vi "Test Multiple Doors API.vi"() -> ()   [LabVIEW 2018]
uses:
  DoorInterface_interface/DoorInterface.lvclass
  Door/Door.lvclass
  Timed Door.lvclass
  Set Target Time (seconds).vi
panel:
  out "error out":errorcluster
  in  "Create New Door":bool
  in  "Door Type":enum32{"Door", "Timed Door"}(radio)
  in  "Timed Door Target Time (seconds)":dbl=5.0
  in  "Door Switches":enum32{"Open Door", "Close Door"}[](array[radio])
  out "Doors":u16[](array[ring])
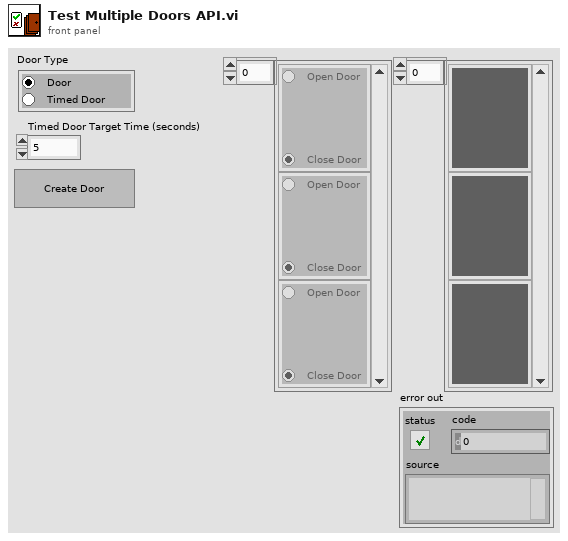
[diagram p1: front panel]
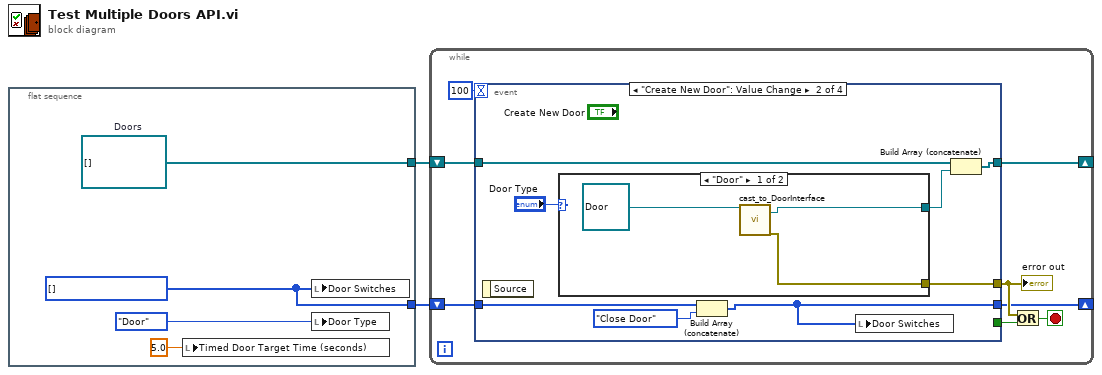
[diagram p0: block diagram]
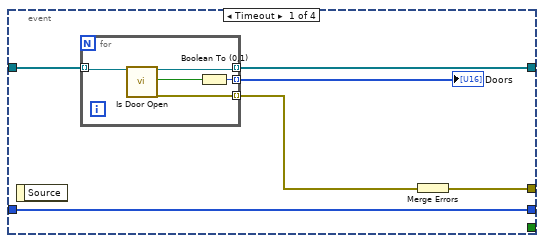
[diagram p2: hidden frame]
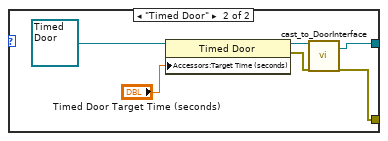
[diagram p3: hidden frame]
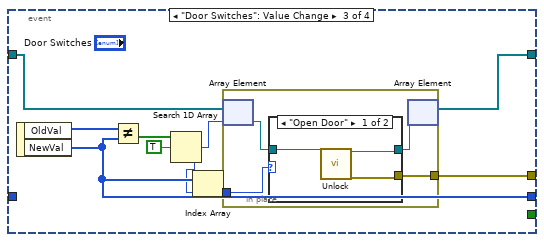
[diagram p4: hidden frame]
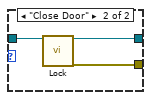
[diagram p5: hidden frame]
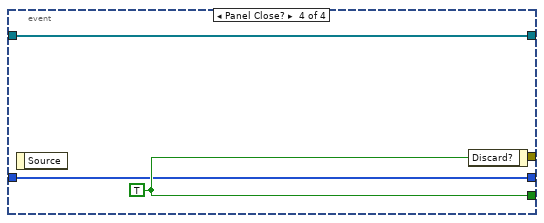
[diagram p6: hidden frame]
diagram:
  n1 = flat-sequence {
    tunnel: [w6] -> w2
    tunnel: [w3] -> w1
    frame #0 {
      w6 = refnum<class "DoorInterface.lvclass">[] []  # Doors
      w3 = enum32{"Open Door", "Close Door"}[] [] items=["Open Door", "Close Door"] ("Door Switch")
      n2 = local write "Timed Door Target Time (seconds)"(5.0 ("Timed Door Target Time (seconds)")) -> ()
      n3 = local write "Door Switches"(w3) -> ()
      n4 = local write "Door Type"(enum32{"Door", "Timed Door"}."Door" ("Door Type")) -> ()
    }
  }
  n5 = while {
    shift-right: [w10] -> _
    shift-left: w2 -> [w12]
    shift-right: [w8] -> _
    shift-left: w1 -> [w9]
    stop <- w7 stop-if-true
    n6 = event shown="[1] \"Create New Door\": Value Change" {
      selector: _ -> [_ _ _ _]
      dyn-events: _ -> [_ _ _ _]
      timeout: 100 -> [_ _ _ _]
      tunnel: w12 -> [w18 w33 w47 w63]
      tunnel: [_ _ _ w64] -> w11
      tunnel: [w19 w32 w48 w63] -> w10
      tunnel: w9 -> [w17 w29 _ w62]
      tunnel: [w17 w27 w46 w62] -> w8
      tunnel: [w15 w26 w43 _] -> w14
      event Timeout {
        n7 = event-data() -> ()  [unwired: 1 in, 1 out]
        n8 = for {
          tunnel: [w25] -> w20 mode=indexing
          tunnel: [w23] -> w19 mode=indexing
          tunnel: w18 -> [w24] mode=indexing
          tunnel: [w22] -> w16 mode=indexing
          n9 = call "Is Door Open.vi"("Interface_object in"=w24) -> ("Interface_object out"=w23:refnum<class "DoorInterface.lvclass">, "Is Door Open?"=w21:bool, "error out"=w22:errorcluster)  [unwired: 16 in]
          n10 = Boolean To (0,1)(Boolean=w21) -> (0, 1=w25:i16)
        }
        "Doors" <- w20
        n11 = Merge Errors(w16) -> (w15:errorcluster)
      }
      event "Create New Door": Value Change {
        n12 = event-data() -> ()  [unwired: 1 in, 1 out]
        n13 = case shown="\"Door\"" "Door Type" {
          tunnel: [w35 w37] -> w30
          tunnel: [w34 w39] -> w26
          frame "Door" {
            n14 = call "cast_to_DoorInterface.vi"("Object in"=refnum<class "Door.lvclass"> refnum ("Door.lvclass")) -> ("Interface_object out"=w35:refnum<class "DoorInterface.lvclass">, "error out"=w34:errorcluster)  [unwired: 17 in]
          }
          frame "Timed Door" {
            n15 = property class="Timed Door"(reference=refnum<class "Timed Door.lvclass"> refnum ("Timed Door.lvclass"), "Accessors:Target Time (seconds)"="Timed Door Target Time (seconds)") -> (reference out=w38:refnum<class "Timed Door.lvclass">, error out=w40:errorcluster)  [unwired: 1 in]
            n16 = call "cast_to_DoorInterface.vi"("Object in"=w38, "error in (no error)"=w40) -> ("Interface_object out"=w37:refnum<class "DoorInterface.lvclass">, "error out"=w39:errorcluster)  [unwired: 16 in]
          }
        }
        n17 = Build Array (concatenate)(w29, enum32{"Open Door", "Close Door"}."Close Door" ("Door Switch")) -> (w27:enum32{"Open Door", "Close Door"}[])
        n18 = local write "Door Switches"(w27) -> ()
        n19 = Build Array (concatenate)(w33, w30) -> (w32:refnum<class "DoorInterface.lvclass">[])
      }
      event "Door Switches": Value Change {
        n20 = event-data() -> ("OldVal"=w51:enum32{"Open Door", "Close Door"}[], "NewVal"=w46:enum32{"Open Door", "Close Door"}[])  [unwired: 1 in]
        n21 = Not Equal?(x=w51, y=w46) -> (x != y?=w50:bool[])
        n22 = Search 1D Array(1D array=w50, element=TRUE) -> (index of element=w45:i32)  [unwired: 1 in]
        n23 = Index Array(array=w46, index=w45) -> (element=w44:enum32{"Open Door", "Close Door"})
        n24 = in-place {
          in-place-border: w44 -> [w53]
          in-place-border: [w52] -> w43
          n25 = in-place-array #1(w47, w45) -> (w55:refnum<class "DoorInterface.lvclass">)
          n26 = case shown="\"Open Door\"" w53 {
            tunnel: w55 -> [w58 w61]
            tunnel: [w57 w60] -> w54
            tunnel: [w56 w59] -> w52
            frame "Open Door" {
              n27 = call "Unlock.vi"("Interface_object in"=w58) -> ("Interface_object out"=w57:refnum<class "DoorInterface.lvclass">, "error out"=w56:errorcluster)  [unwired: 17 in]
            }
            frame "Close Door" {
              n28 = call "Lock.vi"("Interface_object in"=w61) -> ("Interface_object out"=w60:refnum<class "DoorInterface.lvclass">, "error out"=w59:errorcluster)  [unwired: 17 in]
            }
          }
          n29 = in-place-array #1(w54) -> (w48:refnum<class "DoorInterface.lvclass">[])  [unwired: 1 out]
        }
      }
      event Panel Close? {
        w64 = TRUE ("Discard?")
        n30 = event-data() -> ()  [unwired: 1 in, 1 out]
        n31 = event-data("Discard?"=w64) -> ()  [unwired: 1 in, 1 out]
      }
    }
    "error out" <- w14
    n32 = Or(x=w14, y=w11) -> (x .or. y?=w7:bool)
  }
